vi "Truck Custom Probe.vi"(1 "truck":refnum<class "Truck.lvclass">) -> (0 "Boolean":bool)   [LabVIEW 2023, in "Truck.lvclass"]
doc: "A custom probe for the class \"Truck.\" By using this probe, you can view selected data members even if the class is locked."
uses:
  Truck.lvclass
  Truck.lvclass/Truck.ctl
panel:
  out "Bed cargo capacity":dbl format="%#.9f"
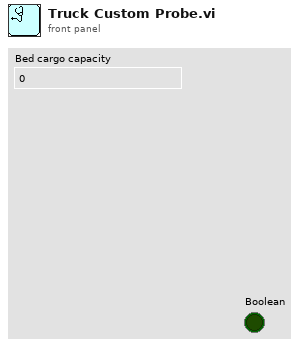
[diagram p1: front panel]
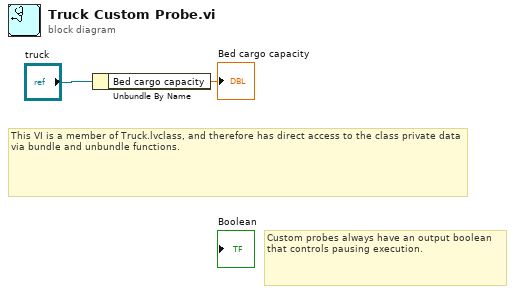
[diagram p0: block diagram]
diagram:
  # "Custom probes always have an output boolean that controls pausing execution."
  # "This VI is a member of Truck.lvclass, and therefore has direct access to the class private data via bundle and unbundle functions."
  n1 = Unbundle By Name("truck") -> ("Bed cargo capacity"=→"Bed cargo capacity":dbl)
